vi "MOKO_Grafic_stm.vi"(8 "error in":errorcluster, 9 "StateMachineSteps":T1[](array[typedef]) {"STM Graph"."Lines"."Color" format="%x"}, 10 "FNs":enum16{"Back", "Front", "Replace"}(ring), 11 "queue in":refnum<queue>) -> (0 "error out":errorcluster, 3 "queue out":refnum<queue>)   [LabVIEW 2018]
uses:
  MOKO_Grafic_STM.ctl
  MOKO_Grafic_ITEM.ctl
  CTL/STM GRAPH.ctl
  CTL/Graph settings.ctl
  CTL/Line.ctl
  Windows/Settings/View.ctl
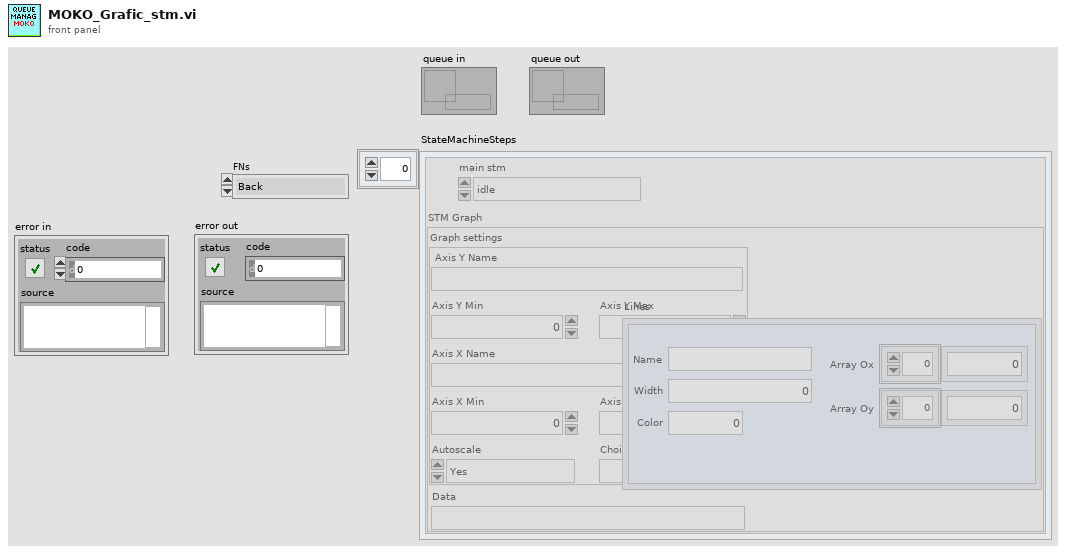
[diagram p1: front panel]
types:
  T1 = typedef "MOKO_Grafic_STM.ctl" = cluster{"main stm":T2, "STM Graph":T3}
  T2 = typedef "MOKO_Grafic_ITEM.ctl" = enum16{"idle", "init", "_____ GRAPH STATE_____ ", "Legend", "Write Graph", "Clear Graph", "close", "Screenshot", "Change Line", "Add Line", "Parse String In", "Add Data", "Change Data", "Graph Settings", "Get Graph Appearance", "Set Graph Appearance", "Delete Data", "Delete Line", "Choose ActPlot", "Set Line Settings", "Increment Smth", "ReWrite Graph", "Autoscale", "Set Autoscale", "Hide Line", "Get Hide Line", "Hide Data", "Show Line", "Get Show Line", "Show Data", "Choose Line", "Change Combo Box", "Send Data", "Receive Data", "Choice Line", "Change Lines", "_____ LED STATE_____ ", "Led Off"}
  T3 = typedef "STM GRAPH.ctl" = cluster{"Graph settings":T4, "Lines":T5[], "Data":string}
  T4 = typedef "Graph settings.ctl" = cluster{"Axis X Min":dbl, "Axis X Name":string, "Axis X Max":dbl, "Axis Y Min":dbl, " Axis Y Name":string, "Axis Y Max":dbl, "Autoscale":enum16{"Yes", "No", "Only Oy", "Only Ox"}, "Choice Line":dbl}
  T5 = typedef "Line.ctl" = cluster{"Width":dbl, "Color":i64, "Array Oy":dbl[], "Array Ox":dbl[], "Name":string, "Plot Visible":T6}
  T6 = typedef "View.ctl" = bool
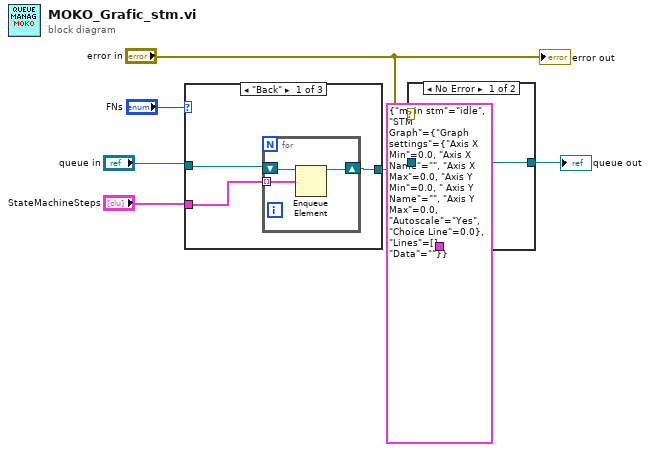
[diagram p0: block diagram]
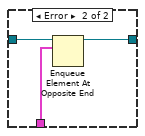
[diagram p2: hidden frame]
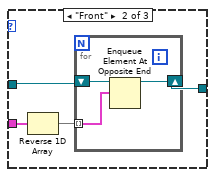
[diagram p3: hidden frame]
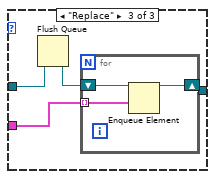
[diagram p4: hidden frame]
diagram:
  n1 = case shown="\"Back\"" "FNs" {
    tunnel: "StateMachineSteps" -> [w8 w14 w22]
    tunnel: "queue in" -> [w10 w16 w24]
    tunnel: [w9 w15 w21] -> w6
    frame "Back" {
      n2 = for {
        shift-right: [w12] -> w9
        shift-left: w10 -> [w13]
        tunnel: w8 -> [w11] mode=indexing
        n3 = Enqueue Element(queue=w13, element=w11) -> (queue out=w12:refnum<queue>)  [unwired: 2 in, 2 out]
      }
    }
    frame "Front" {
      n4 = Reverse 1D Array(array=w14) -> (reversed array=w17:T1[])
      n5 = for {
        tunnel: w17 -> [w19] mode=indexing
        shift-right: [w18] -> w15
        shift-left: w16 -> [w20]
        n6 = Enqueue Element At Opposite End(queue=w20, element=w19) -> (queue out=w18:refnum<queue>)  [unwired: 2 in, 2 out]
      }
    }
    frame "Replace" {
      n7 = Flush Queue(queue=w24) -> (queue out=w23:refnum<queue>)  [unwired: 1 in, 2 out]
      n8 = for {
        tunnel: w22 -> [w26] mode=indexing
        shift-right: [w25] -> w21
        shift-left: w23 -> [w27]
        n9 = Enqueue Element(queue=w27, element=w26) -> (queue out=w25:refnum<queue>)  [unwired: 2 in, 2 out]
      }
    }
  }
  n10 = case shown="No Error" "error in" {
    tunnel: w6 -> [w28 w31]
    tunnel: [w28 w30] -> w3
    tunnel: T1 {"main stm"=enum."idle", "STM Graph"={"Graph settings"={"Axis X Min"=0.0, "Axis X Name"="", "Axis X Max"=0.0, "Axis Y Min"=0.0, " Axis Y Name"="", "Axis Y Max"=0.0, "Autoscale"=enum."Yes", "Choice Line"=0.0}, "Lines"=[], "Data"=""}} ("element") -> [_ w29]
    frame No Error {
    }
    frame Error {
      n11 = Enqueue Element At Opposite End(queue=w31, element=w29) -> (queue out=w30:refnum<queue>)  [unwired: 2 in, 2 out]
    }
  }
  "queue out" <- w3
  "error out" <- "error in"
